vi "Test Load PCX (Memory).vi"(8 "error in (no error)":errorcluster) -> (0 "error out":errorcluster, 3 "Pass?":bool)   [LabVIEW 2020]
uses:
  G-Image/Image IO/Polymorphic VIs/Load Image (Memory).vi
  G-Image/G-Image.lvlib
panel:
  out "Array":cluster{string, "new picture":picture}[](array[cluster])
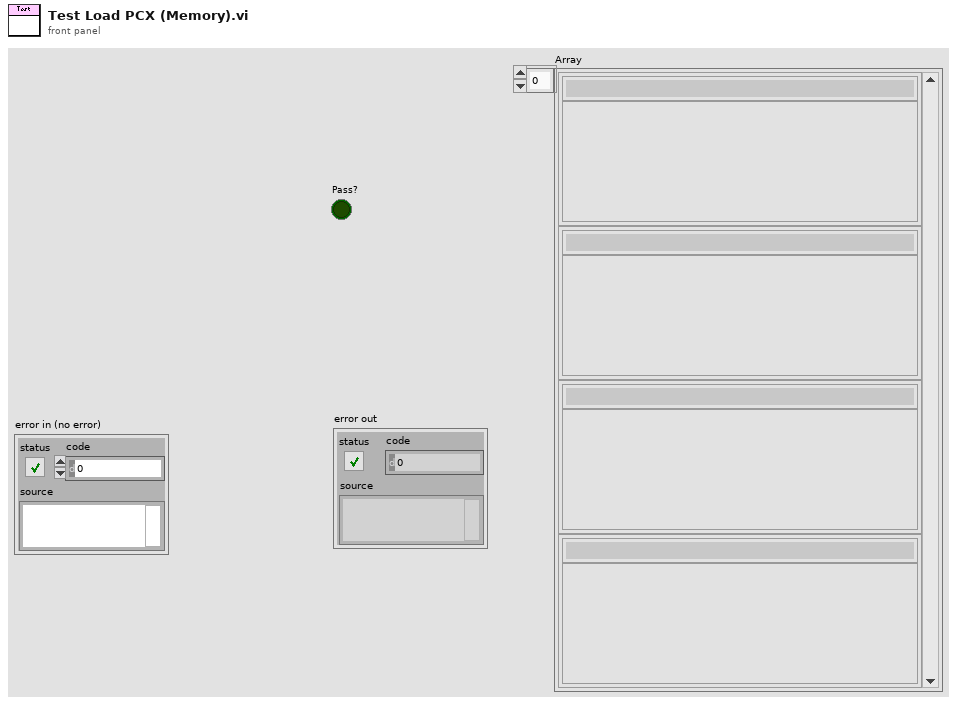
[diagram p1: front panel]
types:
  T1 = typedef "imagedata.ctl" = cluster{"image type":i32, "image depth":i32, "image":u8[], "mask":u8[], "colors":u32[], "Rectangle":cluster{"left":i16, "top":i16, "right":i16, "bottom":i16}}
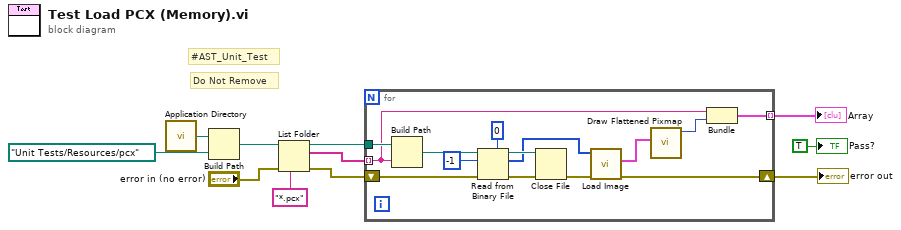
[diagram p0: block diagram]
diagram:
  # "Do Not Remove"
  # "#AST_Unit_Test"
  n1 = call <vilib>:"Application Directory.vi"() -> ("Application Directory"=w11:path)
  n2 = Build Path(base path=w11, name or relative path=path "Unit Tests/Resources/pcx" ("Path")) -> (appended path=w9:path)
  n3 = List Folder(path=w9, pattern="*.pcx", error in="error in (no error)") -> (path out=w7:path, filenames=w6:string[], error out=w4:errorcluster)  [unwired: 1 in, 1 out]
  n4 = for {
    tunnel: w7 -> [w25]
    tunnel: w6 -> [w21] mode=indexing
    shift-right: [w24] -> w3
    shift-left: w4 -> [w18]
    tunnel: [w20] -> w2 mode=indexing
    n5 = Build Path(base path=w25, name or relative path=w21) -> (appended path=w19:path)
    n6 = Read from Binary File(5:u8 0, 8:w18, 10:-1 ("count (1)"), 11:w19) -> (0:w16:errorcluster, 2:w12:u8[], 3:w15:refnum<file>)  [unwired: 2 in, 1 out]
    n7 = Close File(refnum=w15, error in=w16) -> (error out=w14:errorcluster)  [unwired: 1 out]
    n8 = call-poly "Load Image.vi"("error in (no error)"=w14, "Encoded Image"=w12) -> ("error out"=w24:errorcluster, "Image"=w23:T1)  [unwired: 8 in]
    n9 = call <vilib>:"Draw Flattened Pixmap.vi"("image data"=w23) -> ("new picture"=w22:picture)  [unwired: 8 in]
    n10 = Bundle(w21, "new picture"=w22) -> (w20:cluster{string, "new picture":picture})  [unwired: 1 in]
  }
  "error out" <- w3
  "Array" <- w2
  "Pass?" <- TRUE ("Pass?")
